vi "StrictFollower SetControl.vi"(0 "DeviceReference":T1, 1 "StopSendingOtherRequests":bool=TRUE, 2 "MasterID":i32, 7 "error in":errorcluster, 18 "Update Frequency (Hz)":dbl=100.0) -> (20 "DeviceReference Out":T1, 27 "error out":errorcluster)   [LabVIEW 2023]
doc: "Follow the motor output of another Talon while ignoring the master's invert setting.\nIf Talon is in torque control, the torque is copied - which will increase the total torque applied. If Talon is in percent supply output control, the duty cycle is matched. Motor direction is strictly determined by the configured invert and not the master. If you want motor direction to match or oppose the master, use FollowerRequest instead."
uses:
  Users/test.DESKTOP-CORY/Documents/PhoenixProLabVIEWGeneration/CopyDown/DeviceReference.ctl
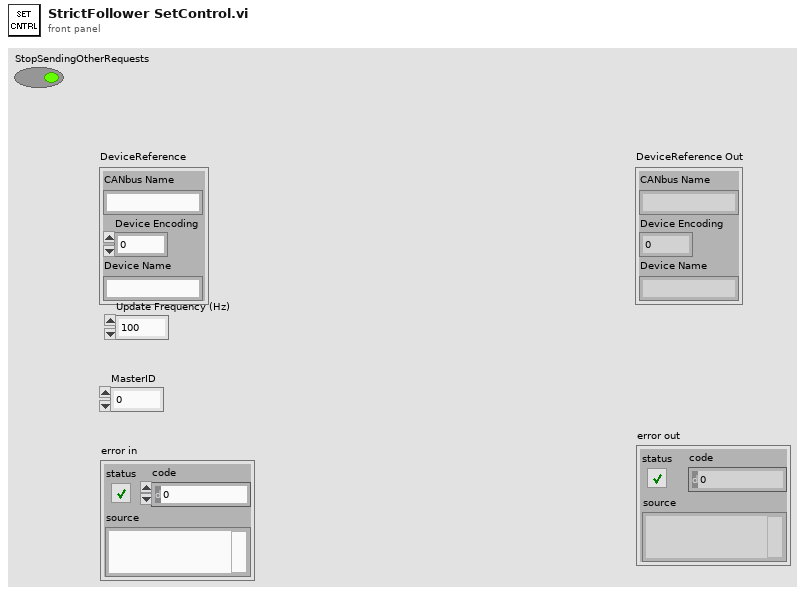
[diagram p1: front panel]
types:
  T1 = typedef "DeviceReference.ctl" = cluster{"CANbus Name":string, "Device Encoding":u32, "Device Name":string}
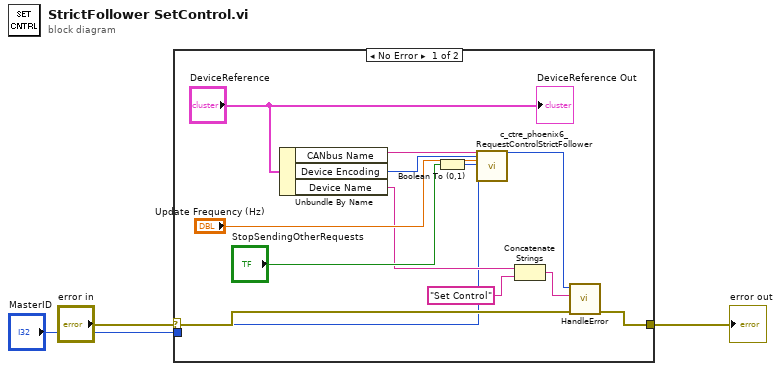
[diagram p0: block diagram]
diagram:
  n1 = case shown="No Error" "error in" {
    selector: "error in" -> [w9 w17]
    tunnel: [w8 w17] -> w2
    tunnel: "MasterID" -> [w4 _]
    frame No Error {
      n2 = Unbundle By Name("DeviceReference") -> ("CANbus Name"=w15:string, "Device Encoding"=w14:u32, "Device Name"=w7:string)
      n3 = Boolean To (0,1)(Boolean="StopSendingOtherRequests") -> (0, 1=w11:i16)
      n4 = call <vilib>:"c_ctre_phoenix6_RequestControlStrictFollower.vi"("String 2"=w15, "Numeric 2"=w14, "Numeric 3"="Update Frequency (Hz)", "Numeric 4"=w11, 4:w4) -> ("Numeric"=w10:i32)  [unwired: 21 in, 1 out]
      n5 = Concatenate Strings(w7, "Set Control" ("origin")) -> (w5:string)
      n6 = call "HandleError.vi"("error in"=w9, "origin"=w5, "Status"=w10) -> ("error out"=w8:errorcluster)  [unwired: 8 in]
      "DeviceReference Out" <- "DeviceReference"
    }
    frame Error {
    }
  }
  "error out" <- w2
